vi "msgDetailsToJSON.vi"(8 "error in (no error)":errorcluster, 10 "msgData":T1={"msgName"="move", "msgDetails"="\"tolerance\":2,"}, 11 "TcpServerBase in":refnum<class "TcpServerBase.lvclass">) -> (0 "error out":errorcluster, 2 "JSON string":string, 3 "TcpServerBase out":refnum<class "TcpServerBase.lvclass">)   [LabVIEW 2018, in "TcpServerBase.lvclass"]
doc: "Convert the message name and message detailes into JSON string, to be sent to TCP Client."
uses:
  TcpServerBase.lvclass
  typedef/msgTypeDef.ctl
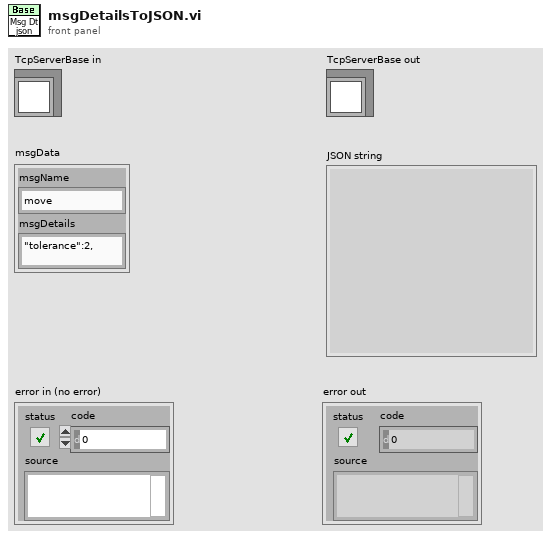
[diagram p1: front panel]
types:
  T1 = typedef "TcpServerBase.lvclass/msgTypeDef.ctl" = cluster{"msgName":string, "msgDetails":string}
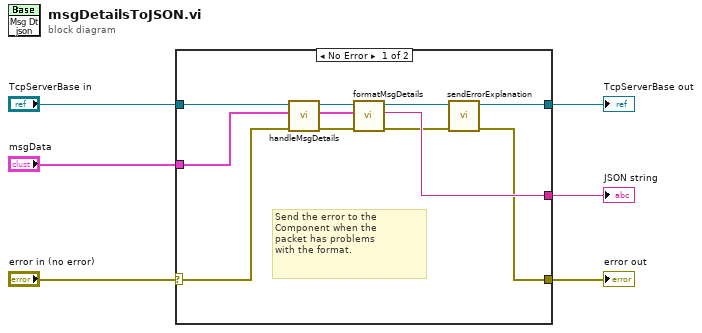
[diagram p0: block diagram]
diagram:
  n1 = case shown="No Error" "error in (no error)" {
    selector: "error in (no error)" -> [w13 w18]
    tunnel: "TcpServerBase in" -> [w16 w19]
    tunnel: [w7 w19] -> w5
    tunnel: [w14 _] -> w4
    tunnel: [w9 w18] -> w2
    tunnel: "msgData" -> [w11 _]
    frame No Error {
      # "Send the error to the\nComponent when the\npacket has problems\nwith the format."
      n2 = call "handleMsgDetails.vi"("error in (no error)"=w13, "msgTypeDef"=w11, "TcpServerBase in"=w16) -> ("error out"=w17:errorcluster, "msgTypeDef"=w10:T1, "TcpServerBase out"=w15:refnum<class "TcpServerBase.lvclass">)  [unwired: 6 in]
      n3 = call "formatMsgDetails.vi"("error in (no error)"=w17, "msgCluster"=w10, "TcpServerBase in"=w15) -> ("error out"=w12:errorcluster, "jsonString"=w14:string, "TcpServerBase out"=w8:refnum<class "TcpServerBase.lvclass">)  [unwired: 6 in]
      n4 = call "sendErrorExplanation.vi"("error in (no error)"=w12, "TcpServerBase in"=w8) -> ("error out"=w9:errorcluster, "TcpServerBase out"=w7:refnum<class "TcpServerBase.lvclass">)  [unwired: 8 in]
    }
    frame Error {
    }
  }
  "JSON string" <- w4
  "TcpServerBase out" <- w5
  "error out" <- w2
